vi "Unicode String Probe (All).vi"(11 "String":string) -> (2 "Value String":string, 3 "Boolean":bool)   [LabVIEW 2020]
uses:
  Unicode/Controls/String Encoding.ctl
  Private/Conversion/Text to UTF-8.vi
  Private/Conversion/Polymorphic VIs/Text to UTF-8 (LabVIEW String).vi
  Private/Conversion/Encoded UTF-8 String to Encoded UTF-16LE String.vi
  Unicode/SubVIs/UTF-16 Byte Swap.vi
  Private/Conversion/UTF-8 to Text.vi
  Private/Conversion/Polymorphic VIs/UTF-8 to Text (LabVIEW String).vi
  Private/Conversion/Encoded UTF-16LE String to Encoded UTF-8 String.vi
  Unicode/SubVIs/Byte Order Marks.vi
  G-Unicode.lvlib
panel:
  out "Input Length":i32
  out "Truncated":bool
  out "ANSI":string
  out "UTF-16BE":string
  out "UTF-16LE":string
  out "UTF-8":string
  out "Byte Order Mark":bool
  out "Detected Encoding":T1
  out "Raw Bytes":u8[](array[numeric]) format="%02x"
  out "Raw String":string
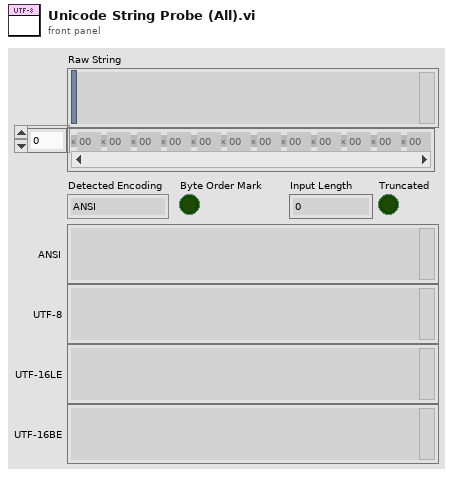
[diagram p1: front panel]
types:
  T1 = typedef "G-Unicode.lvlib/String Encoding.ctl" = enum16{"ANSI", "UTF-8", "UTF-16LE", "UTF-16BE", "Unknown"}
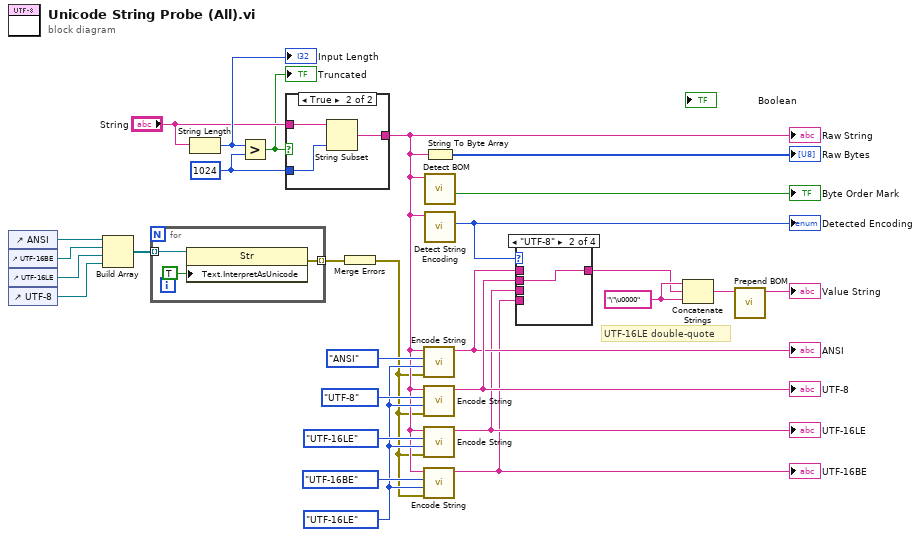
[diagram p0: block diagram]
diagram:
  w3 = "\"\u0000" ("string")
  w8 = 1024 ("y")
  w19 = String_Encoding."UTF-16LE" ("Output Encoding (UTF-8)")
  # "UTF-16LE double-quote"
  n1 = control-ref of="ANSI"() -> (w18:refnum<vi>)
  n2 = control-ref of="UTF-16BE"() -> (w17:refnum<vi>)
  n3 = control-ref of="UTF-16LE"() -> (w16:refnum<vi>)
  n4 = control-ref of="UTF-8"() -> (w15:refnum<vi>)
  n5 = Build Array(w18, w17, w16, w15) -> (w14:refnum<vi>[])
  n6 = for {
    tunnel: w14 -> [w31] mode=indexing
    tunnel: [w29] -> w13 mode=indexing
    n7 = property on="Property Node" class="Str"(reference=w31, "Text.InterpretAsUnicode"=TRUE ("Text.Interpret As Unicode")) -> (error out=w29:errorcluster)  [unwired: 1 in, 1 out]
  }
  n8 = String Length(string="String") -> (length=w9:i32)
  "Input Length" <- w9
  n9 = Greater?(x=w9, y=w8) -> (0:w4:bool)
  "Truncated" <- w4
  n10 = case shown="True" w4 {
    tunnel: "String" -> [w32 w35]
    tunnel: w8 -> [_ w34]
    tunnel: [w32 w33] -> w7
    frame False {
    }
    frame True {
      n11 = String Subset(string=w35, length (rest)=w34) -> (substring=w33:string)  [unwired: 1 in]
    }
  }
  "Raw String" <- w7
  n12 = Merge Errors(w13) -> (w5:errorcluster)
  n13 = call "Encode String.vi"("error in"=w5, "Output Encoding (UTF-16LE)"=w19, "Input Encoding (ANSI)"=String_Encoding."ANSI", "String in"=w7) -> ("String out"=w12:string)  [unwired: 6 in, 1 out]
  "ANSI" <- w12
  n14 = call "Encode String.vi"("error in"=w5, "Output Encoding (UTF-16LE)"=w19, "Input Encoding (ANSI)"=String_Encoding."UTF-8", "String in"=w7) -> ("String out"=w21:string)  [unwired: 6 in, 1 out]
  "UTF-8" <- w21
  n15 = call "Encode String.vi"("error in"=w5, "Output Encoding (UTF-16LE)"=w19, "Input Encoding (ANSI)"=String_Encoding."UTF-16LE", "String in"=w7) -> ("String out"=w11:string)  [unwired: 6 in, 1 out]
  "UTF-16LE" <- w11
  n16 = call "Encode String.vi"("error in"=w5, "Output Encoding (UTF-16LE)"=w19, "Input Encoding (ANSI)"=String_Encoding."UTF-16BE", "String in"=w7) -> ("String out"=w10:string)  [unwired: 6 in, 1 out]
  "UTF-16BE" <- w10
  n17 = String To Byte Array(string=w7) -> (unsigned byte array=→"Raw Bytes":u8[])
  n18 = call "Detect BOM.vi"("String"=w7) -> ("BOM Found"=→"Byte Order Mark":bool)  [unwired: 9 in, 1 out]
  n19 = call "Detect String Encoding.vi"("String"=w7) -> ("Encoding"=w24:T1)  [unwired: 8 in, 2 out]
  "Detected Encoding" <- w24
  n20 = case shown="\"UTF-8\"" w24 {
    tunnel: w21 -> [_ w37 _ _]
    tunnel: [w36 w37 w38 w39] -> w1
    tunnel: w11 -> [_ _ w38 _]
    tunnel: w10 -> [_ _ _ w39]
    tunnel: w12 -> [w36 _ _ _]
    frame "ANSI", Default {
    }
    frame "UTF-8" {
    }
    frame "UTF-16LE" {
    }
    frame "UTF-16BE" {
    }
  }
  n21 = Concatenate Strings(w3, w1, w3) -> (w2:string)
  n22 = call "Prepend BOM.vi"("String"=w2) -> ("String with BOM"=→"Value String":string)  [unwired: 9 in, 1 out]
